vi "nanocal manage curvature plot.vi"(6 "hist size":i32=25, 7 "aggregator action":T6, 9 "xyz IN":T5) -> (0 "fit OUT":dbl[](array[numeric]), 1 "xyz OUT":T5, 2 "output cluster":T3, 3 "arrays OUT":T4)   [LabVIEW 2020]
uses:
  agregator -- action.ctl
  <vilib>/Analysis/Matrix/Datatypes/RealMatrix.ctl
  <vilib>/Analysis/Matrix/Datatypes/ComplexMatrix.ctl
  interpolation state - real.ctl
  array -- fit control .ctl
  linear interpolation - real -- V2.vi
  <vilib>/Analysis/Matrix/NI_Matrix.lvlib
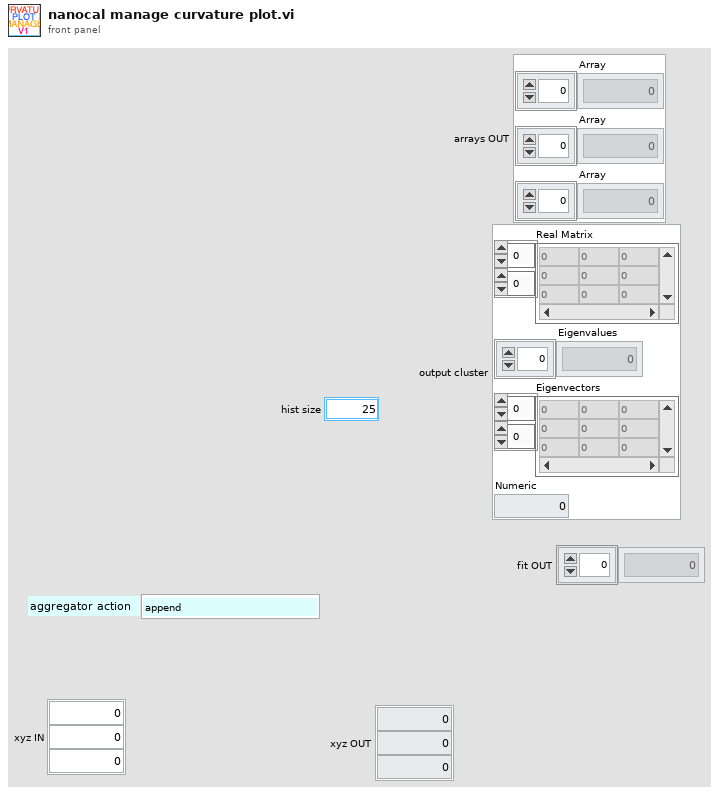
[diagram p1: front panel]
types:
  T1 = typedef "NI_Matrix.lvlib/RealMatrix.ctl" = dbl[][]
  T2 = typedef "NI_Matrix.lvlib/ComplexMatrix.ctl" = cdb[][]
  T3 = cluster{"Real Matrix":T1, "Eigenvalues":cdb[], "Eigenvectors":T2, "Numeric":cdb}
  T4 = cluster{"Array ":dbl[], "Array ":dbl[], "Array ":dbl[]}
  T5 = cluster{"Numeric":dbl, "Numeric":dbl, "Numeric":dbl}
  T6 = typedef "agregator -- action.ctl" = enum16{"append", "interpolate", "empty!", "force", "init", "scale", "read last"}
  T7 = typedef "interpolation state - real.ctl" = cluster{"Array ":dbl[], "actual size":i32, "requested size":i32}
  T8 = typedef "array -- fit control .ctl" = enum16{"fit", "calc", "check", "init"}
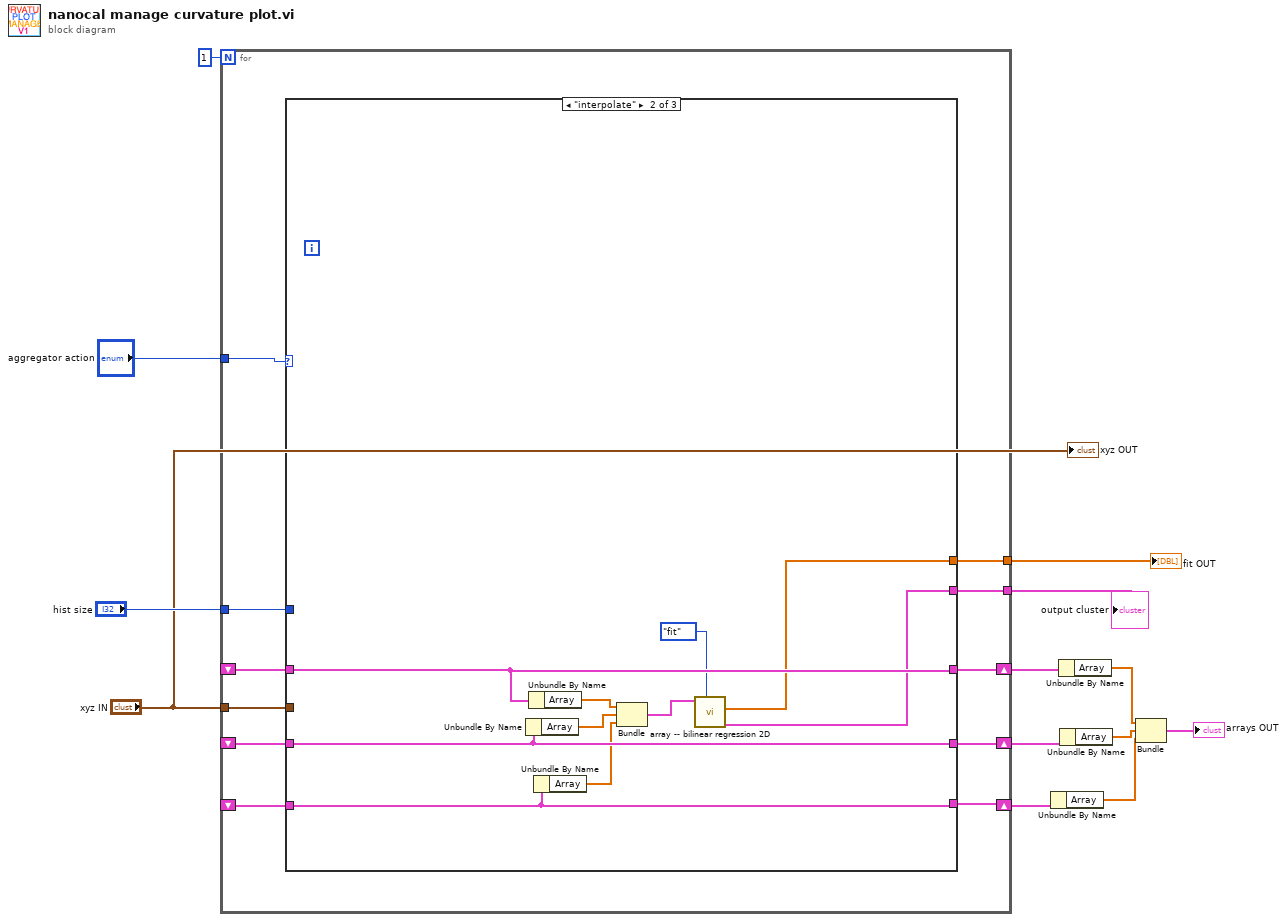
[diagram p0: block diagram]
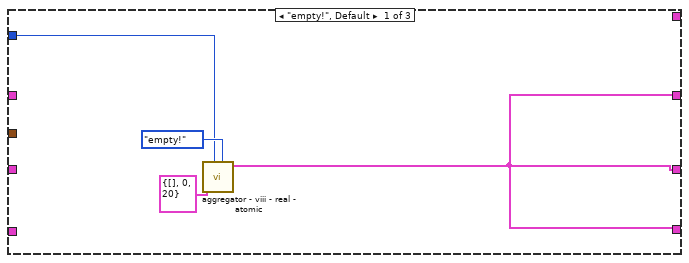
[diagram p2: hidden frame]
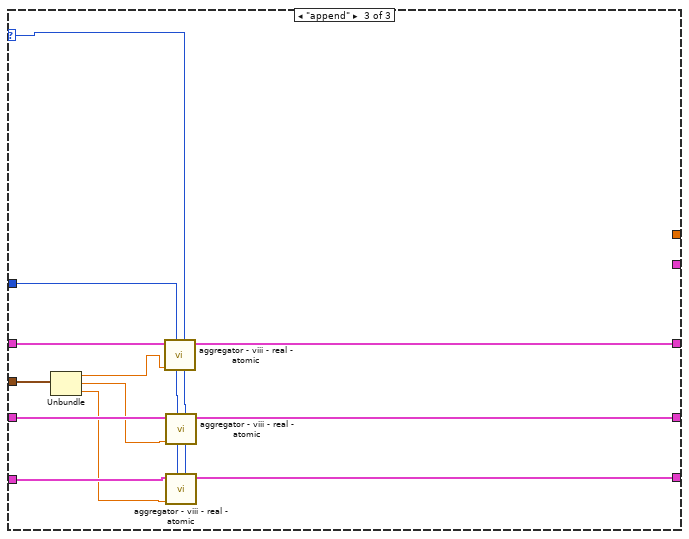
[diagram p3: hidden frame]
diagram:
  n1 = for {
    N: 1 -> [_]
    shift-right: [w22] -> w9
    shift-left: _ -> [w19]
    shift-right: [w23] -> w10
    shift-left: _ -> [w24]
    tunnel: "hist size" -> [w21]
    tunnel: "aggregator action" -> [w20]
    shift-right: [w18] -> w8
    shift-left: _ -> [w17]
    tunnel: "xyz IN" -> [w16]
    tunnel: [w15] -> w3
    tunnel: [w14] -> w2
    n2 = case shown="\"interpolate\"" w20 {
      selector: w20 -> [_ _ w44]
      tunnel: w24 -> [_ w38 w50]
      tunnel: [w25 w38 w49] -> w23
      tunnel: [w25 w37 w48] -> w22
      tunnel: w21 -> [w26 _ w43]
      tunnel: w19 -> [_ w37 w47]
      tunnel: [w25 w36 w46] -> w18
      tunnel: w17 -> [_ w36 w45]
      tunnel: w16 -> [_ _ w42]
      tunnel: [_ w30 _] -> w15
      tunnel: [_ w29 _] -> w14
      frame "empty!", Default {
        n3 = call "aggregator - viii - real - atomic.vi"("aggregator action"=agregator_--_action."empty!", "requested size"=w26, "state IN"=T7 {"Array "=[], "actual size"=0, "requested size"=20}) -> ("state OUT"=w25:T7)  [unwired: 5 in, 3 out]
      }
      frame "interpolate" {
        n4 = Unbundle By Name(w37) -> ("Array"=w34:dbl[])
        n5 = Unbundle By Name(w38) -> ("Array"=w35:dbl[])
        n6 = Unbundle By Name(w36) -> ("Array"=w33:dbl[])
        n7 = Bundle("Array"=w35, "Array"=w34, "Array"=w33) -> (w32:T4)  [unwired: 1 in]
        n8 = call "array -- bilinear regression 2D.vi"("action"=array_--_fit_control_."fit", "xyz IN"=w32) -> ("output cluster"=w29:T3, "fit OUT"=w30:dbl[])  [unwired: 6 in, 2 out]
      }
      frame "append" {
        n9 = Unbundle(w42) -> ("Numeric"=w41:dbl, "Numeric"=w40:dbl, "Numeric"=w39:dbl)
        n10 = call "aggregator - viii - real - atomic.vi"("aggregator action"=w44, "requested size"=w43, "number"=w41, "state IN"=w50) -> ("state OUT"=w49:T7)  [unwired: 4 in, 3 out]
        n11 = call "aggregator - viii - real - atomic.vi"("aggregator action"=w44, "requested size"=w43, "number"=w40, "state IN"=w47) -> ("state OUT"=w48:T7)  [unwired: 4 in, 3 out]
        n12 = call "aggregator - viii - real - atomic.vi"("aggregator action"=w44, "requested size"=w43, "number"=w39, "state IN"=w45) -> ("state OUT"=w46:T7)  [unwired: 4 in, 3 out]
      }
    }
  }
  "fit OUT" <- w3
  "output cluster" <- w2
  n13 = Unbundle By Name(w8) -> ("Array"=w5:dbl[])
  n14 = Unbundle By Name(w10) -> ("Array"=w7:dbl[])
  n15 = Unbundle By Name(w9) -> ("Array"=w6:dbl[])
  n16 = Bundle("Array"=w7, "Array"=w6, "Array"=w5) -> (→"arrays OUT":T4)  [unwired: 1 in]
  "xyz OUT" <- "xyz IN"
